vi "Get Self.vi"(11 "Addresses in":refnum<class "Addresses.lvclass">) -> (2 "Self":refnum<class "Msg Type Strategy.lvclass">)   [LabVIEW 2021, in "jettl.lvlib" / "Addresses.lvlib" / "Addresses.lvclass"]
uses:
  Addresses.lvclass
  Addresses.lvclass/Addresses.ctl
  Msg Type Strategy/Msg Type Strategy/Msg Type Strategy.lvclass
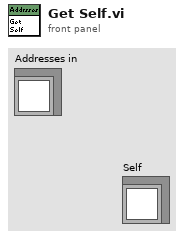
[diagram p1: front panel]
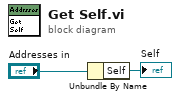
[diagram p0: block diagram]
diagram:
  n1 = Unbundle By Name("Addresses in") -> ("Self"=→"Self":refnum<class "Msg Type Strategy.lvclass">)
